vi "Test Suite from LVLib.vi"(8 "error in (no error)":errorcluster, 11 "Test Case In":refnum<class "LUnit Test Suite Tests.lvclass">) -> (0 "error out":errorcluster, 3 "Test Case Out":refnum<class "LUnit Test Suite Tests.lvclass">)   [LabVIEW 2020, in "LUnit Test Suite Tests.lvclass"]
uses:
  LUnit Test Suite Tests.lvclass
  C:/Program Files (x86)/National Instruments/LabVIEW 2020/vi.lib/Astemes/LUnit/Test Case.lvclass
  Result/Type.ctl
  <vilib>/Astemes/LUnit/Test Case.lvclass/Test Case.ctl
  b74e4934-f044-4222-b3dd-fc90e6c1bd4f.vi
  <vilib>/Astemes/LUnit/Palette/Pass.vi
  <vilib>/Astemes/LUnit/Palette/Fail.vi
  <vilib>/Astemes/LUnit/Compare Variants.vi
  <vilib>/Astemes/LUnit/Describe Comparison.vi
  <vilib>/Astemes/LUnit/Set Assertion Type.vi
  <vilib>/Astemes/LUnit/Add test result.vi
  <vilib>/Astemes/LUnit/Variant to string.vi
  <vilib>/Astemes/LUnit/LUnit Record Assertion Result.vi
  <vilib>/Astemes/LUnit/LUnit Aggregate Assertion Results.vi
  <vilib>/Astemes/LUnit/Method Result/LUnit Merge Status.vi
  <vilib>/Astemes/LUnit/LUnit Concatenate result strings.vi
  Mock Result Observer/Mock Result Observer.lvclass
  C:/Git/astemes-lunit/source/Rewrite Project/Result Observer/Result Observer.lvclass
  <vilib>/Utility/Data Type/Get Type Information.vi
  <vilib>/Utility/LVClass/Get LV Class Name.vi
  LUnit Test Suite/LUnit Test Suite V2.lvclass
  Result/Result.lvlib
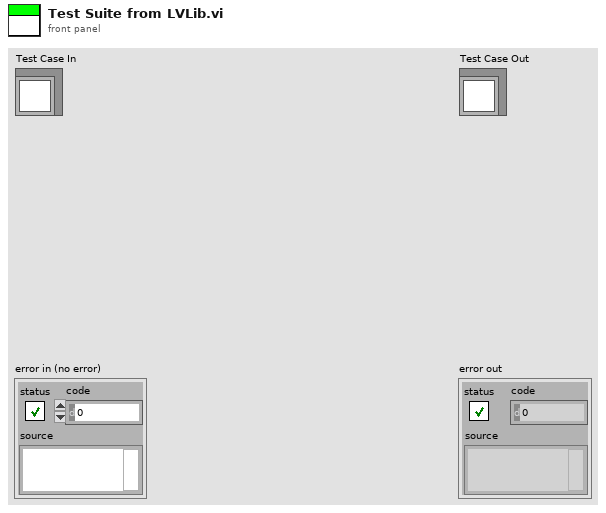
[diagram p1: front panel]
types:
  T1 = typedef "Result.lvlib/Type.ctl" = enum16{"Method", "Case", "Suite", "Pass", "Fail", "Skip", "Pass if", "Fail if", "Pass if Error", "Fail if Error", "Pass if Equal", "Fail if Equal"}
  T2 = typedef "Result.lvlib/Result.ctl" = cluster{"Name":string, "Message":string, "Description":string, "Status":T3, "Result Type":T1, "Execution Time":dbl}
  T3 = typedef "Result.lvlib/Status.ctl" = enum16{"", "Passed", "Failed", "Error", "Skipped", "Setup Error", "Broken", "Teardown Error"}
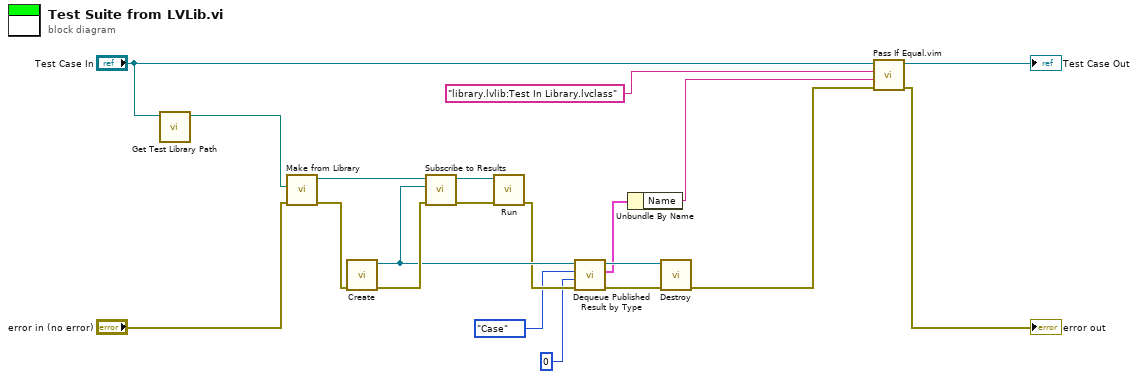
[diagram p0: block diagram]
diagram:
  n1 = call "Get Test Library Path.vi"("LUnit Test Suite Tests in"="Test Case In") -> ("lvlib path"=w17:path)  [unwired: 9 in, 1 out]
  n2 = call "Make from Library.vi"("error in (no error)"="error in (no error)", "Library Path"=w17) -> ("error out"=w12:errorcluster, "LUnit Test Suite V2 Out"=w15:refnum<class "LUnit Test Suite V2.lvclass">)  [unwired: 8 in]
  n3 = call "Create.vi"("error in (no error)"=w12) -> ("error out"=w13:errorcluster, "Mock Result Observer out"=w11:refnum<class "Mock Result Observer.lvclass">)  [unwired: 9 in]
  n4 = call-dynamic "Subscribe to Results.vi"("error in (no error)"=w13, "Result Observer"=w11, "LUnit Test Suite V2 In"=w15) -> ("error out"=w16:errorcluster, "LUnit Test Suite V2 Out"=w14:refnum<class "LUnit Test Suite V2.lvclass">)  [unwired: 7 in]
  n5 = call-dynamic "Run.vi"("error in (no error)"=w16, "Run in"=w14) -> ("error out"=w10:errorcluster)  [unwired: 8 in, 1 out]
  n6 = call "Dequeue Published Result by Type.vi"("error in (no error)"=w10, "timeout in ms"=0, "Result Type"=Type."Case", "Mock Result Observer In"=w11) -> ("error out"=w6:errorcluster, "Result"=w4:T2, "Mock Result Observer Out"=w9:refnum<class "Mock Result Observer.lvclass">)  [unwired: 4 in, 1 out]
  n7 = Unbundle By Name(w4) -> ("Name"=w3:string)
  n8 = call "Destroy.vi"("error in (no error)"=w6, "Mock Result Observer in"=w9) -> ("error out"=w7:errorcluster)  [unwired: 9 in]
  n9 = call "Pass If Equal.vim"("error in (no error)"=w7, "Actual"=w3, "Expected"="library.lvlib:Test In Library.lvclass" ("class name"), "LUnit Test Case In"="Test Case In") -> ("error out"=→"error out":errorcluster, "LUnit Test Case Out"=→"Test Case Out":refnum<class "LUnit Test Suite Tests.lvclass">)  [unwired: 6 in]
